vi "周期设置.vi"(11 "定时控制输入":T1) -> (3 "定时控制输出":T1)   [LabVIEW 2022 SP3, in "斯坦道多参数.lvlib"]
uses:
  <vilib>/Utility/miscctls.llb/LVPointTypeDef.ctl
panel:
  in  "延时启动时间":u32 caption="延时启动时间："
  in  "确定":bool
  in  "取消":bool
  in  "定时功能启用":bool
  out "选项卡控件":enum32{"定点启动", "间隔启动"}(tab)
  in  "24H周期设置":bool[](xcontrol)
  in  "定时间隔":u32
  in  "周期设置类型":enum16{"定点启动", "间隔启动"}(ring)
  # "周期设置类型："
  # "请输入定时启动间隔"
  # "min"
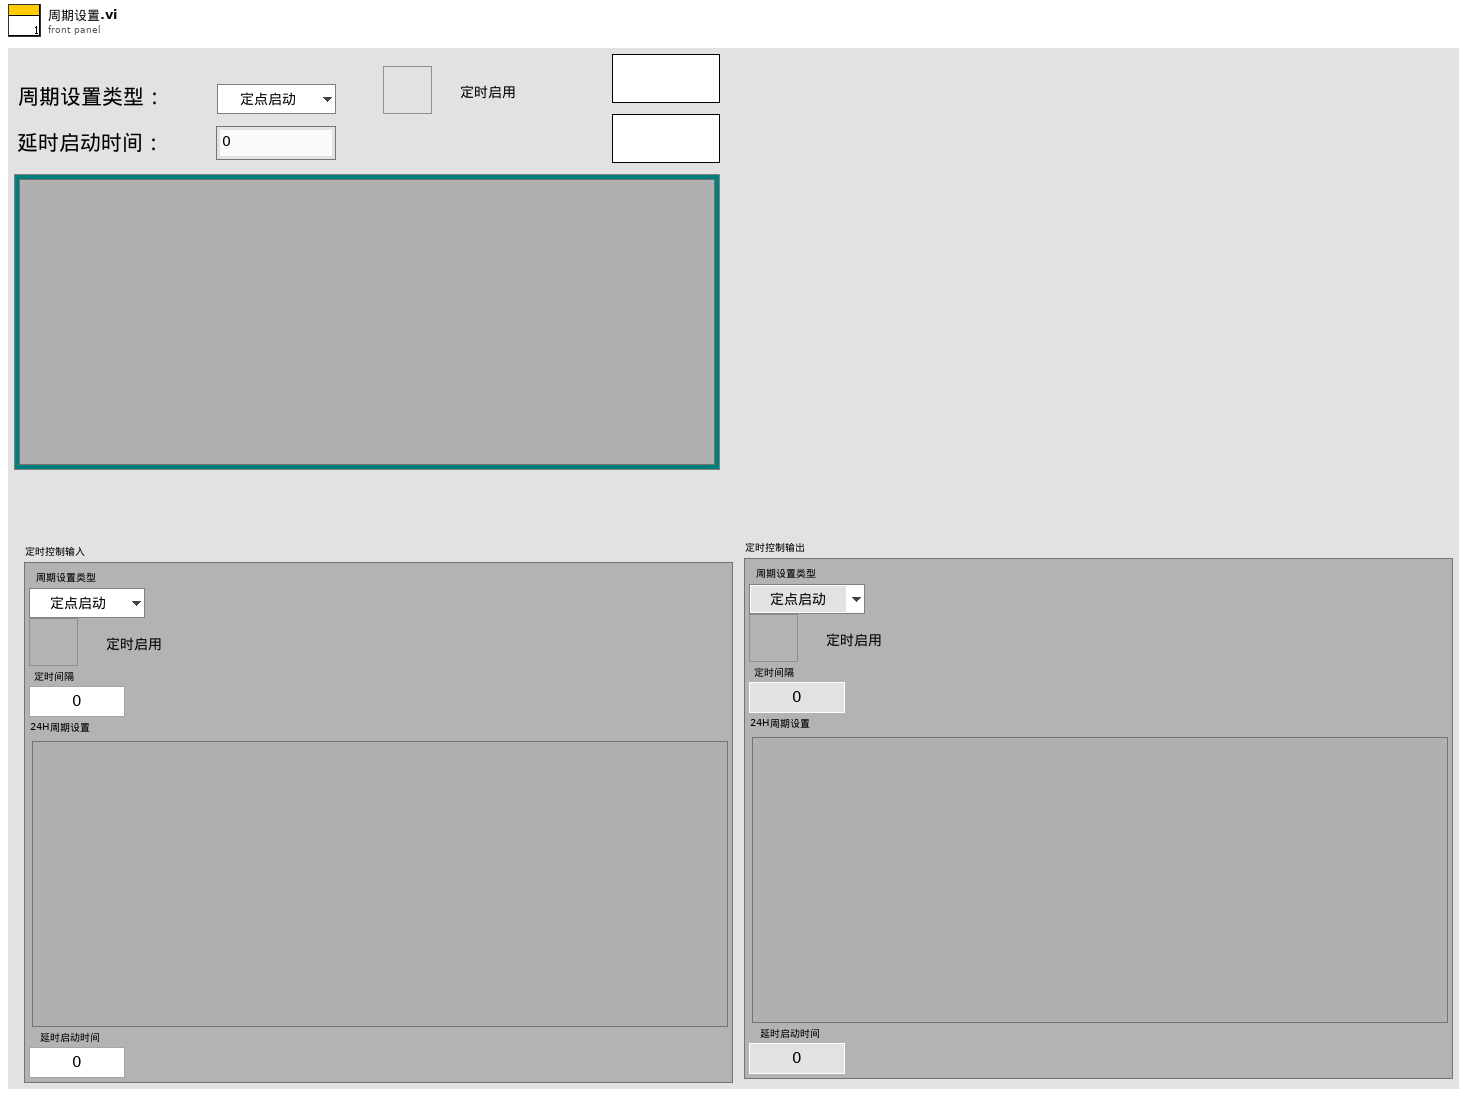
[diagram p1: front panel]
types:
  T1 = cluster{"周期设置类型":enum16{"定点启动", "间隔启动"}, "定时功能启用":bool, "定时间隔":u32, "24H周期设置":bool[], "延时启动时间":u32}
  T2 = typedef "LVPointTypeDef.ctl" = cluster{"Horizontal":i16, "Vertical":i16}
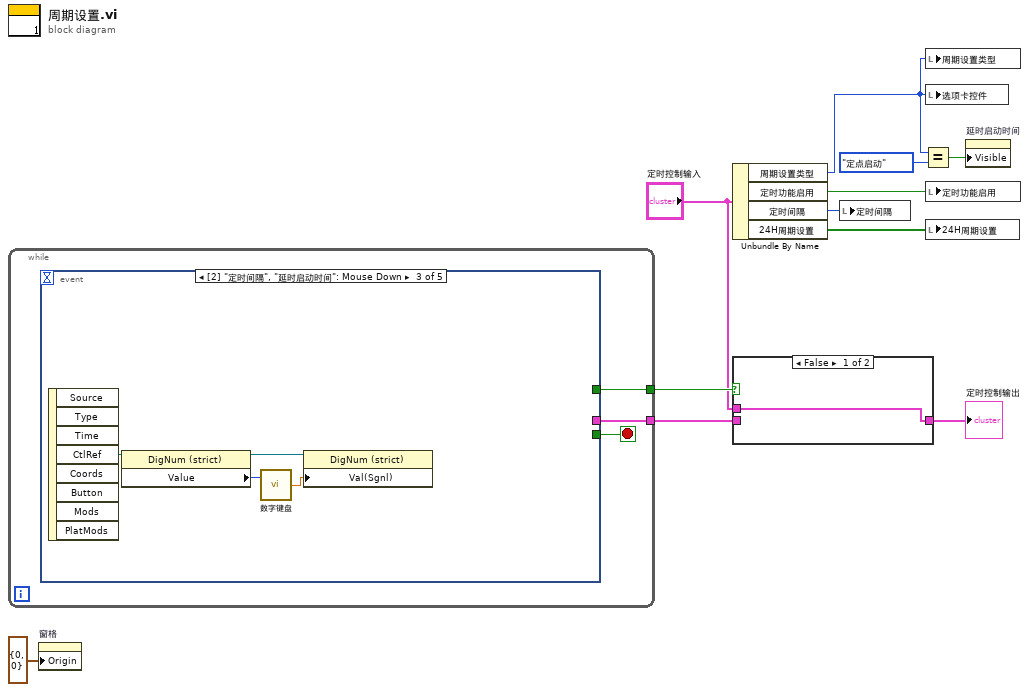
[diagram p0: block diagram]
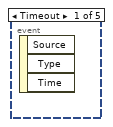
[diagram p3: hidden frame]
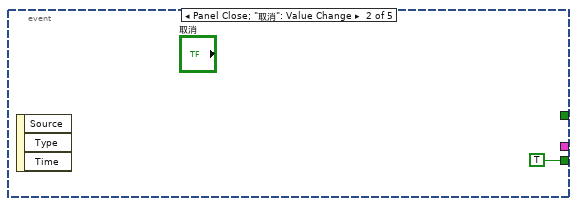
[diagram p4: hidden frame]
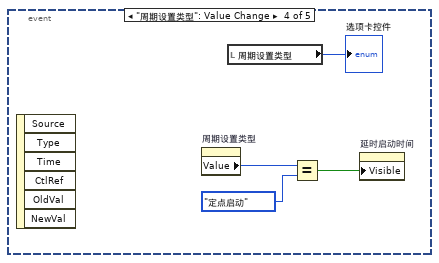
[diagram p5: hidden frame]
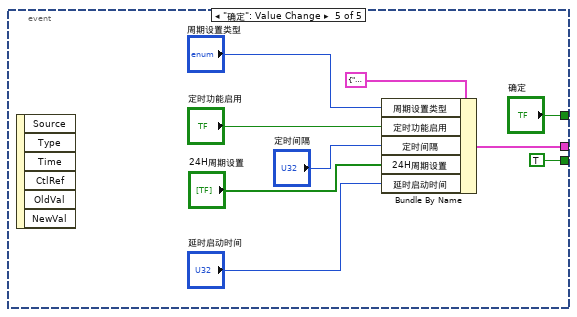
[diagram p6: hidden frame]
diagram:
  n1 = while {
    tunnel: [w13] -> w7
    tunnel: [w12] -> w8
    stop <- w14 stop-if-true
    n2 = event shown="[2] \"定时间隔\", \"延时启动时间\": Mouse Down" {
      selector: _ -> [_ _ _ _ _]
      dyn-events: _ -> [_ _ _ _ _]
      timeout: _ -> [_ _ _ _ _]
      tunnel: [_ TRUE _ _ TRUE] -> w14
      tunnel: [_ _ _ _ w28] -> w13
      tunnel: [_ _ _ _ "确定"] -> w12
      event Timeout {
        n3 = event-data() -> ()  [unwired: 1 in, 3 out]
      }
      event Panel Close; "取消": Value Change {
        n4 = event-data() -> ()  [unwired: 1 in, 3 out]
      }
      event "定时间隔", "延时启动时间": Mouse Down {
        n5 = event-data() -> ("CtlRef"=w19:refnum<vi>)  [unwired: 1 in, 7 out]
        n6 = property class="DigNum (strict)"(reference=w19) -> (reference out=w16:refnum<vi>, "Value"=w18:u32)  [unwired: 1 in, 1 out]
        n7 = call "数字键盘.vi"("OldNumber"=w18) -> ("NewNumber"=w17:dbl)  [unwired: 1 in]
        n8 = property class="DigNum (strict)"(reference=w16, "Val(Sgnl)"=w17) -> ()  [unwired: 1 in, 2 out]
      }
      event "周期设置类型": Value Change {
        n9 = event-data() -> ()  [unwired: 1 in, 6 out]
        n10 = property on="周期设置类型" class="Enum (strict)"() -> ("Value"=w20:enum16{"定点启动", "间隔启动"})  [unwired: 2 in, 2 out]
        n11 = local read "周期设置类型"() -> (→"选项卡控件":enum16{"定点启动", "间隔启动"})
        n12 = Equal?(x=w20, y=enum16{"定点启动", "间隔启动"}."定点启动") -> (x = y?=w22:bool)
        n13 = property on="延时启动时间" class="DigNum (strict)"("Visible"=w22) -> ()  [unwired: 2 in, 2 out]
      }
      event "确定": Value Change {
        n14 = event-data() -> ()  [unwired: 1 in, 6 out]
        n15 = Bundle By Name(cluster=T1 {"周期设置类型"=enum."定点启动", "定时功能启用"=FALSE, "定时间隔"=0, "24H周期设置"=[], "延时启动时间"=0} ("定时控制输入"), "周期设置类型"="周期设置类型", "定时功能启用"="定时功能启用", "定时间隔"="定时间隔", "24H周期设置"="24H周期设置", "延时启动时间"="延时启动时间") -> (w28:T1)
      }
    }
  }
  n16 = property on="窗格" class="Pane"("Origin"=T2 {"Horizontal"=0, "Vertical"=0} ("原点")) -> ()  [unwired: 2 in, 2 out]
  n17 = Unbundle By Name("定时控制输入") -> ("周期设置类型"=w1:enum16{"定点启动", "间隔启动"}, "定时功能启用"=w11:bool, "定时间隔"=w10:u32, "24H周期设置"=w9:bool[])
  n18 = case shown="False" w8 {
    tunnel: w7 -> [_ w34]
    tunnel: [w33 w34] -> w5
    tunnel: "定时控制输入" -> [w33 _]
    frame False {
    }
    frame True {
    }
  }
  "定时控制输出" <- w5
  n19 = local write "定时间隔"(w10) -> ()
  n20 = Equal?(x=w1, y=enum16{"定点启动", "间隔启动"}."定点启动") -> (x = y?=w2:bool)
  n21 = local write "周期设置类型"(w1) -> ()
  n22 = local write "选项卡控件"(w1) -> ()
  n23 = local write "定时功能启用"(w11) -> ()
  n24 = local write "24H周期设置"(w9) -> ()
  n25 = property on="延时启动时间" class="DigNum (strict)"("Visible"=w2) -> ()  [unwired: 2 in, 2 out]
